vi "measure-6221-SR830(SubVI).vi"(9 "config":refnum<queue>, 11 "错误输入":errorcluster) -> (4 "输出数组":string[](array[string]), 8 "错误输出":errorcluster)   [LabVIEW 2019, in "SubVI.lvlib"]
uses:
  SubVI.lvlib
  config.ctl
  Instrument.ctl
  lib/QDInstrument.dll
  lib/Stanford Research 830/Public/Data/Read (All Parameters).vi
  lib/Stanford Research 830/Stanford Research 830.lvlib
  lib/Keithley 622x/Keithley 622x.lvlib
panel:
  out "输出簇":T1={"initialize"="", "6221"={"6221 Resource"="GPIB0::24::INSTR", "Delta status"=FALSE}, "7001"={"Ch"=FALSE}, "SR830+6221"={"source"=0, "阻抗"=0.0, "量程入 4"=0, "量程入 3"=0, "量程入 2"=0, "量程入 1"=0, "电流"=0.0, "SR830 2"=FALSE, "SR830 3"=FALSE, "SR830 4"=FALSE, "SR830 1"=FALSE, "VISA 1"="", "VISA 2"="", "VISA 3"="", "VISA 4"="", "量程"=enum."量程每次测量会判定"}, "2400"={"2400"=FALSE, "VISA"=""}, "ch"={"ch str"="", "ch1"=FALSE, "ch2"=FALSE, "布尔"=FALSE}, "error"=FALSE, "数据文件路径"=path "", "log"={"log路径"=path "", "log interval"=0.0}, "Instrument"={"335 Resource"="GPIB0::24::INSTR", "Input (0:A)"=0, "Instrument Type"=3, "quantum design"=refnum, "Heater Output (1:1)"=1}} {"Instrument"."Input (0:A)" items=["A", "B"]; "Instrument"."Instrument Type" items=["PPMS", "VersaLab", "DynaCool", "SVSM", "Lakeshore335", "PPMS-Rotate"]; "Instrument"."Heater Output (1:1)" items=["1"=1, "2"=2]; "SR830+6221"."source" items=["SR830 1", "SR830 2", "SR830 3", "SR830 4"]}
  # "(真是通道1，假是通道2)"
  # "(真是通道1，假是通道2)"
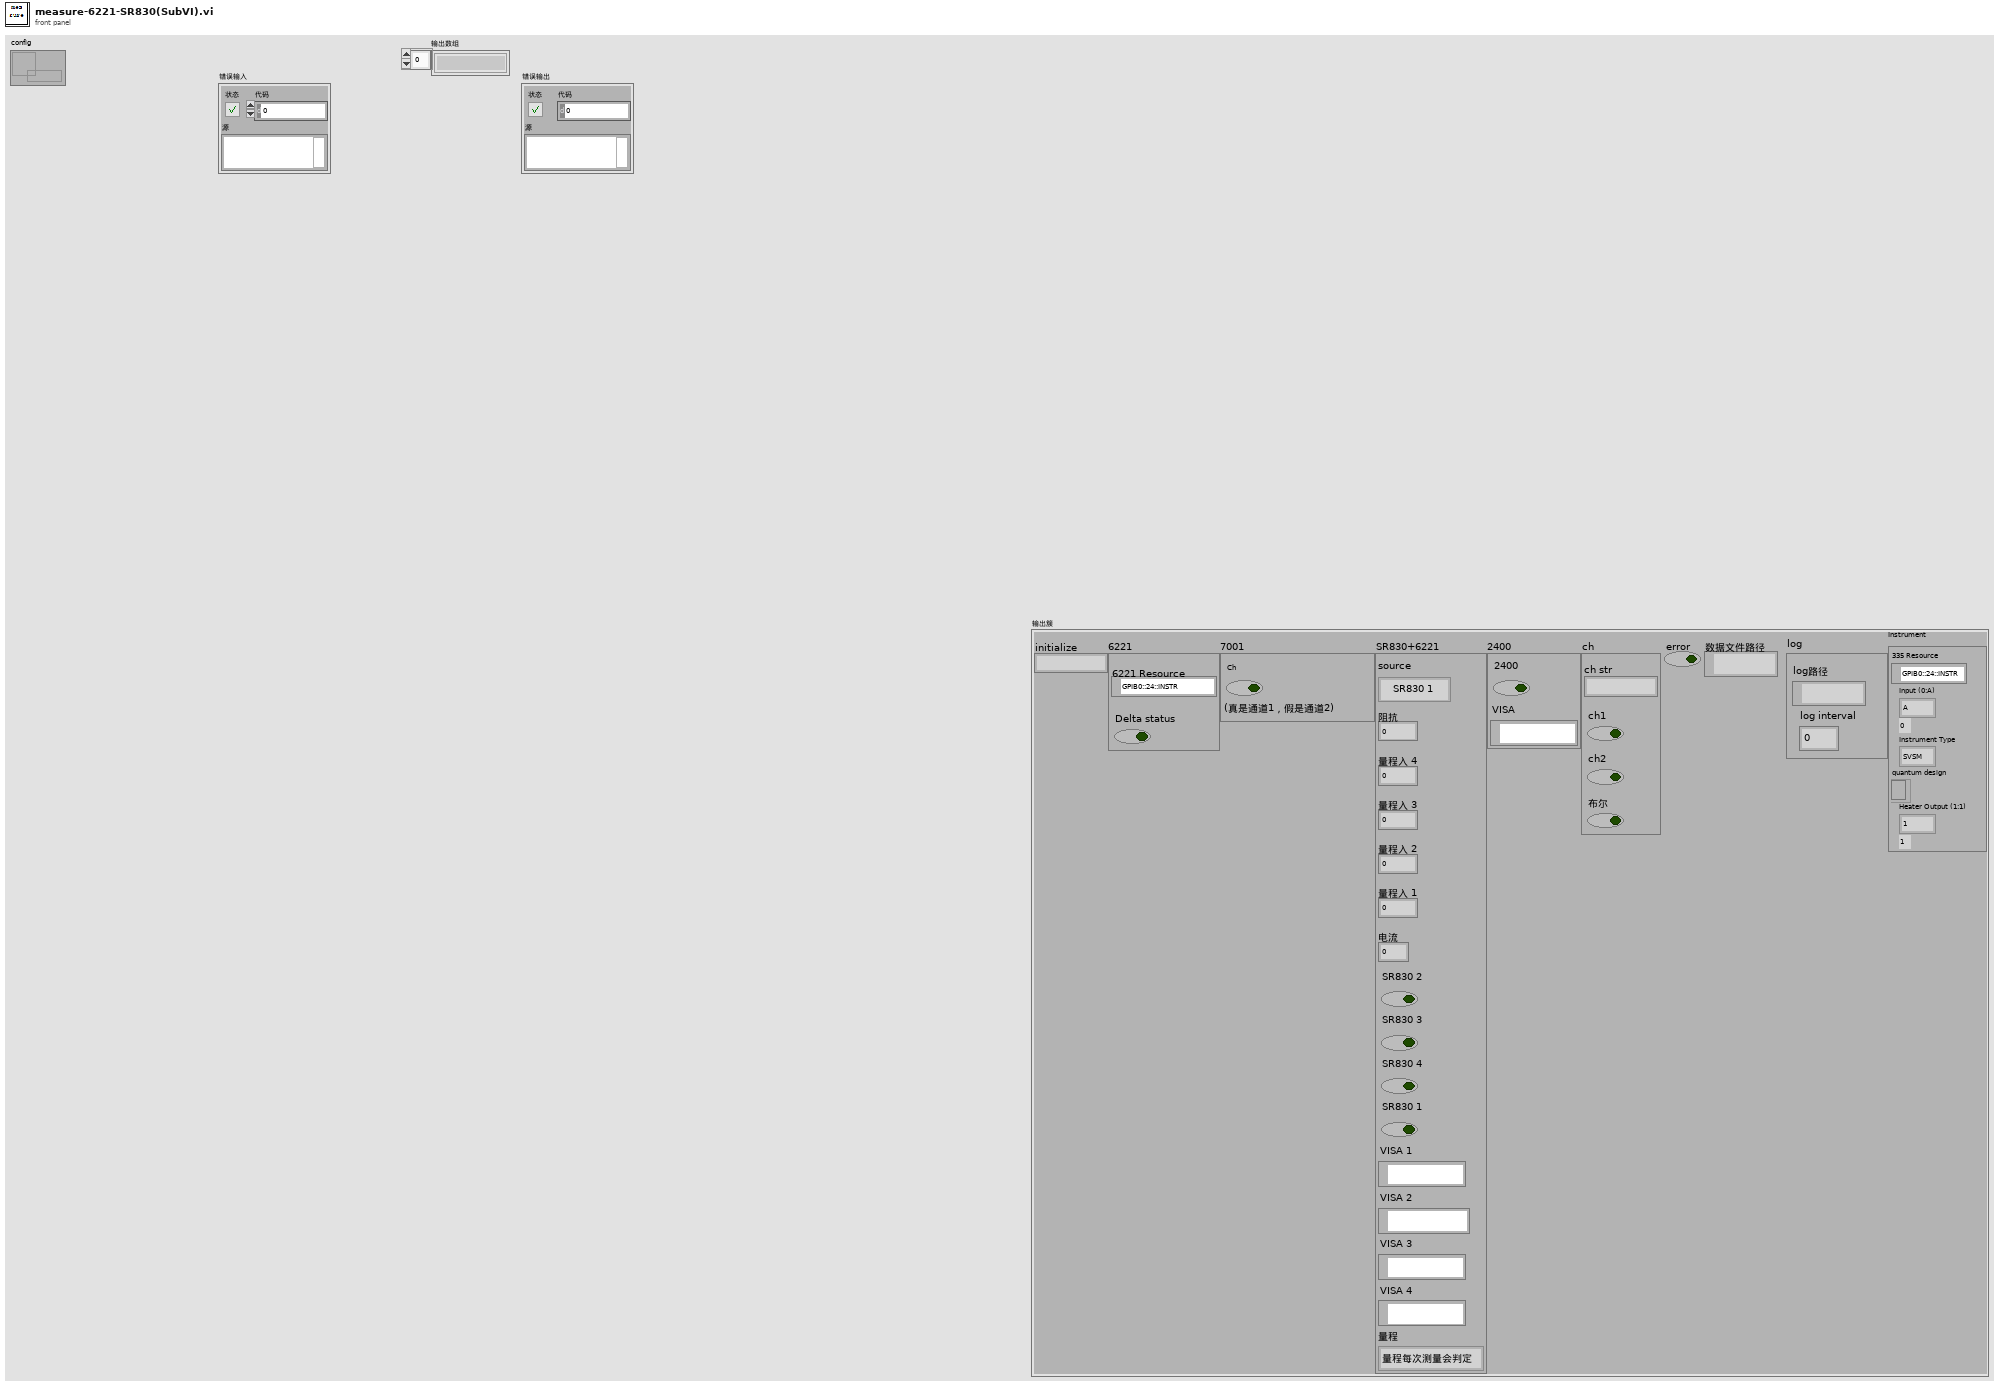
[diagram p1: front panel]
types:
  T1 = typedef "config.ctl" = cluster{"initialize":string, "6221":cluster{"6221 Resource":refnum<visa-resource-name>, "Delta status":bool}, "7001":cluster{"Ch":bool}, "SR830+6221":cluster{"source":u16, "阻抗":dbl, "量程入 4":i32, "量程入 3":i32, "量程入 2":i32, "量程入 1":i32, "电流":dbl, "SR830 2":bool, "SR830 3":bool, "SR830 4":bool, "SR830 1":bool, "VISA 1":refnum<visa-resource-name>, "VISA 2":refnum<visa-resource-name>, "VISA 3":refnum<visa-resource-name>, "VISA 4":refnum<visa-resource-name>, "量程":enum16{"量程每次测量会判定", "量程不变为设定值"}}, "2400":cluster{"2400":bool, "VISA":refnum<visa-resource-name>}, "ch":cluster{"ch str":string, "ch1":bool, "ch2":bool, "布尔":bool}, "error":bool, "数据文件路径":path, "log":cluster{"log路径":path, "log interval":dbl}, "Instrument":T2}
  T2 = typedef "Instrument.ctl" = cluster{"335 Resource":refnum<visa-resource-name>, "Input (0:A)":u16, "Instrument Type":i32, "quantum design":refnum<k24>, "Heater Output (1:1)":u16}
  T3 = cluster{"X-Value":dbl, "Y-Value":dbl, "R-Value":dbl, "Theta-Value":dbl, "Aux In 1 Value":dbl, "Aux In 2 Value":dbl, "Aux In 3 Value":dbl, "Aux In 4 Value":dbl, "Reference Frequency":dbl, "Channel 1 Display":dbl, "Channel 2 Display":dbl}
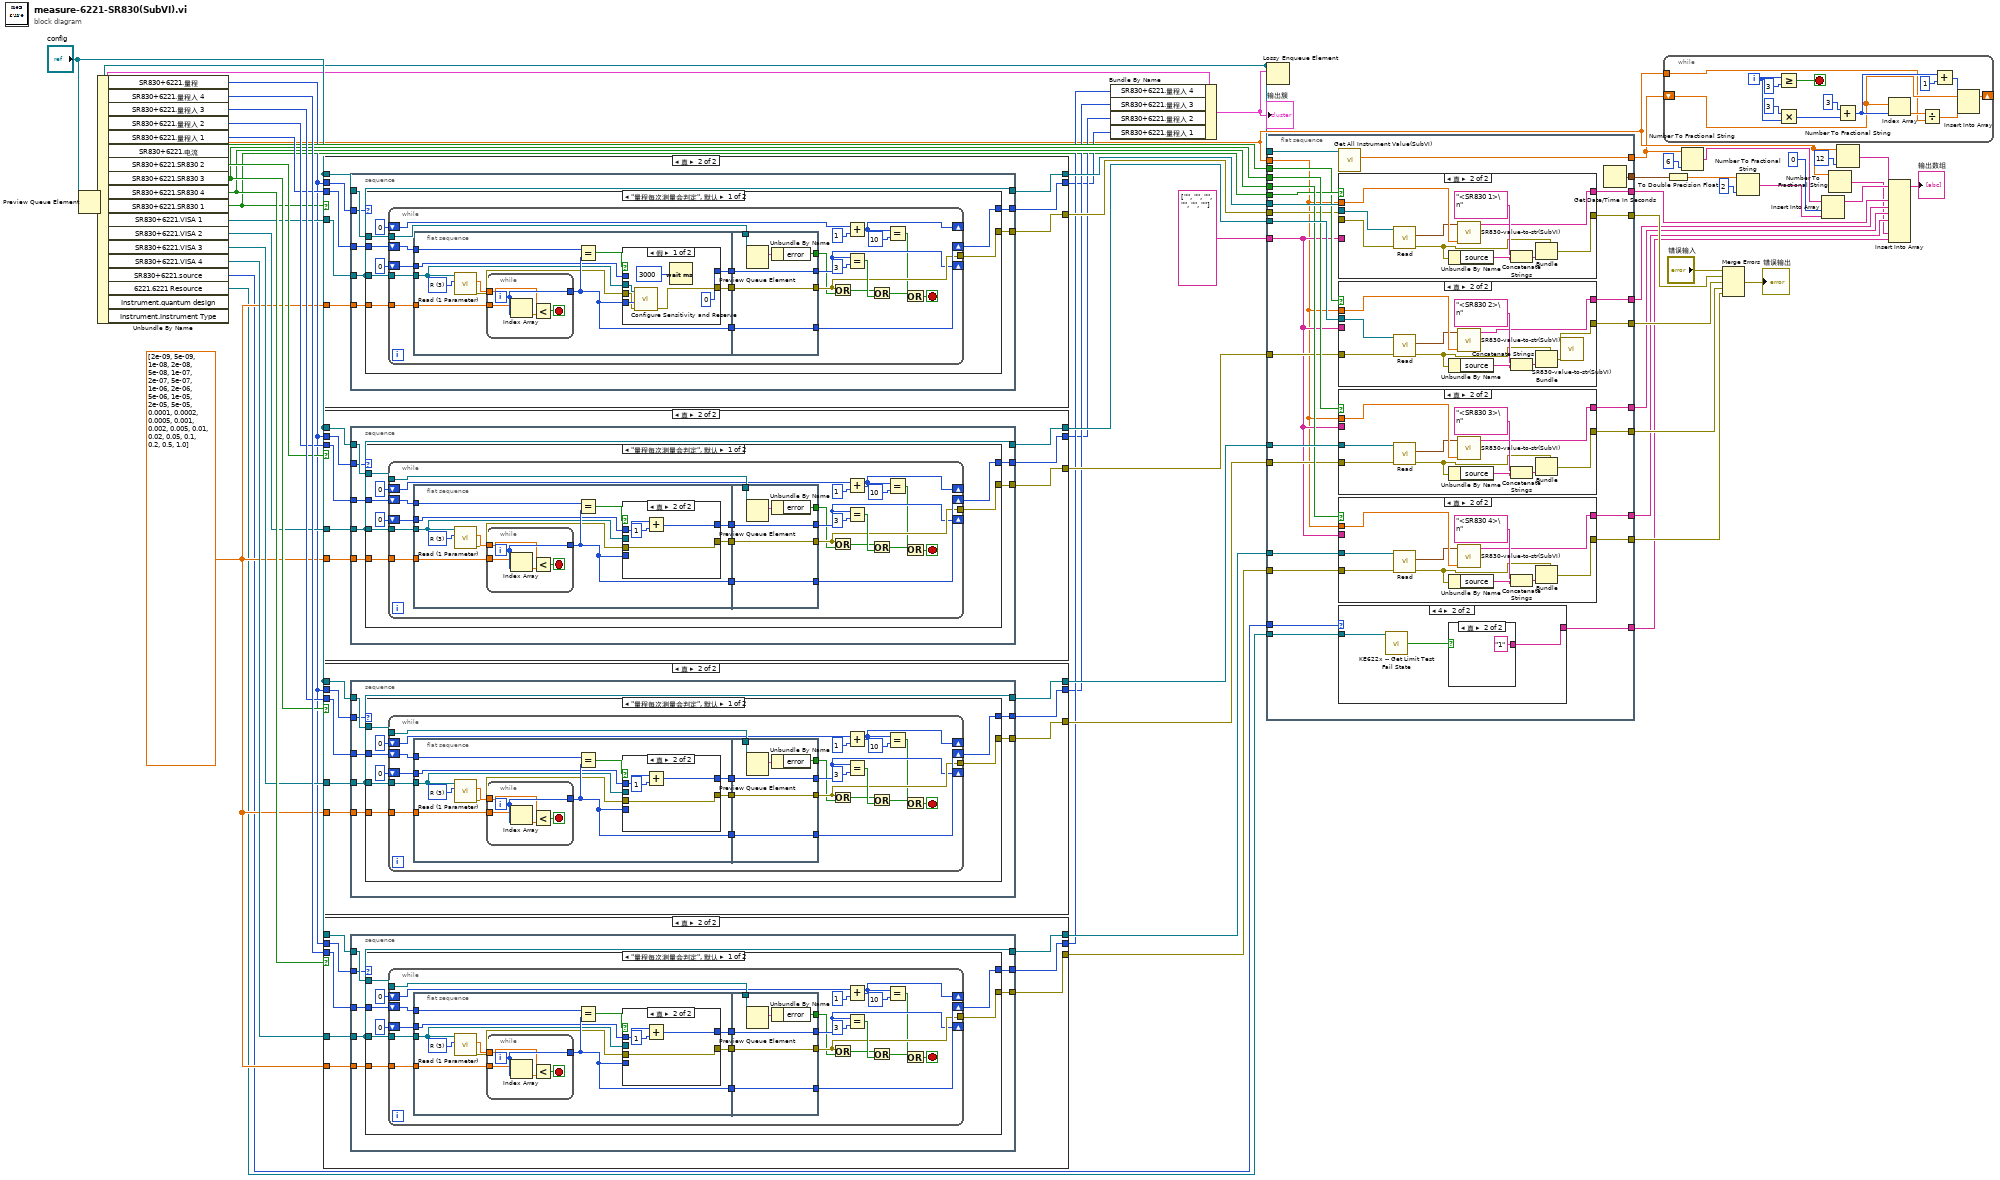
[diagram p0: block diagram]
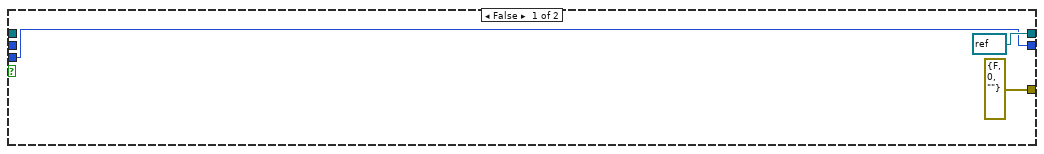
[diagram p2: hidden frame]
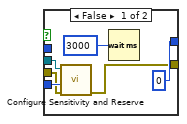
[diagram p3: hidden frame]
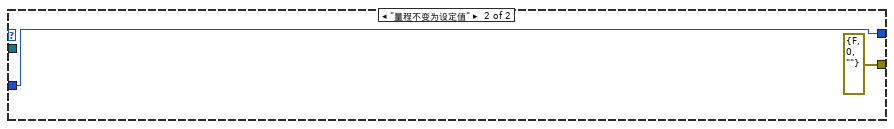
[diagram p4: hidden frame]
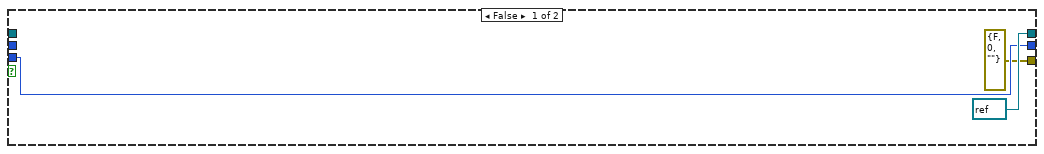
[diagram p5: hidden frame]
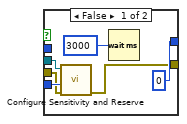
[diagram p6: hidden frame]
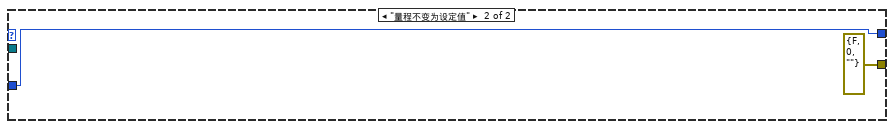
[diagram p7: hidden frame]
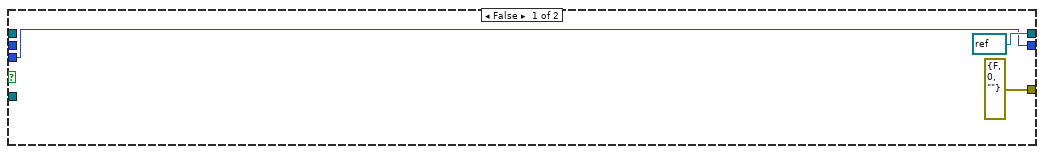
[diagram p8: hidden frame]
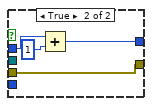
[diagram p9: hidden frame]
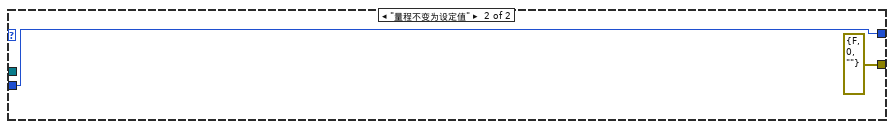
[diagram p10: hidden frame]
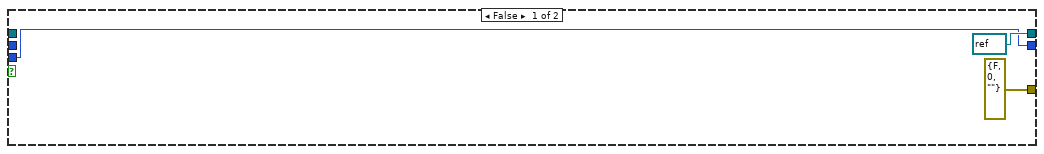
[diagram p11: hidden frame]
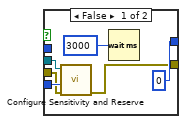
[diagram p12: hidden frame]
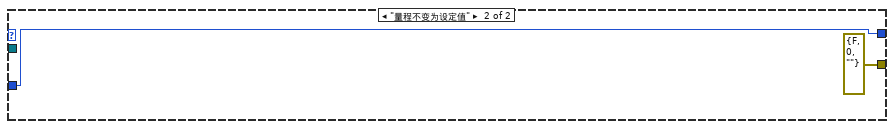
[diagram p13: hidden frame]
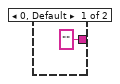
[diagram p14: hidden frame]
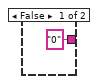
[diagram p15: hidden frame]
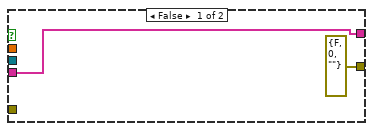
[diagram p16: hidden frame]
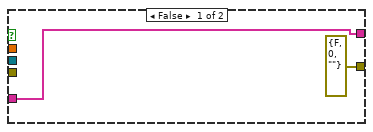
[diagram p17: hidden frame]
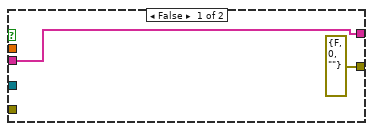
[diagram p18: hidden frame]
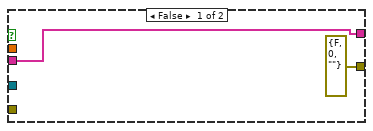
[diagram p19: hidden frame]
diagram:
  w11 = dbl[] [2e-09, 5e-09, 1e-08, 2e-08, 5e-08, 1e-07, 2e-07, 5e-07, 1e-06, 2e-06, 5e-06, 1e-05, 2e-05, 5e-05, 0.0001, 0.0002, 0.0005, 0.001, 0.002, 0.005, 0.01, 0.02, 0.05, 0.1, 0.2, 0.5, 1.0]
  n1 = Preview Queue Element(queue="config") -> (queue out=w2:refnum<queue>, element=w9:T1)  [unwired: 2 in, 2 out]
  n2 = Unbundle By Name(w9) -> ("SR830+6221.量程"=w32:enum16{"量程每次测量会判定", "量程不变为设定值"}, "SR830+6221.量程入 4"=w43:i32, "SR830+6221.量程入 3"=w42:i32, "SR830+6221.量程入 2"=w41:i32, "SR830+6221.量程入 1"=w40:i32, "SR830+6221.电流"=w5:dbl, "SR830+6221.SR830 2"=w39:bool, "SR830+6221.SR830 3"=w38:bool, "SR830+6221.SR830 4"=w37:bool, "SR830+6221.SR830 1"=w19:bool, "SR830+6221.VISA 1"=w36:refnum<visa-resource-name>, "SR830+6221.VISA 2"=w35:refnum<visa-resource-name>, "SR830+6221.VISA 3"=w34:refnum<visa-resource-name>, "SR830+6221.VISA 4"=w33:refnum<visa-resource-name>, "SR830+6221.source"=w7:u16, "6221.6221 Resource"=w6:refnum<visa-resource-name>)  [unwired: 2 out]
  n3 = case shown="真" w19 {
    tunnel: [refnum<visa-resource-name> refnum ("VISA引用句柄输出") w69] -> w56
    tunnel: w32 -> [_ w68]
    tunnel: w36 -> [_ w67]
    tunnel: w40 -> [w60 w66]
    tunnel: [w60 w65] -> w28
    tunnel: "config" -> [_ w64]
    tunnel: [errorcluster {"status"=FALSE, "code"=0, "source"=""} ("error out") w63] -> w53
    tunnel: w11 -> [_ w62]
    frame False {
    }
    frame True {
      n4 = stacked-sequence {
        tunnel: [w75] -> w63
        tunnel: [w71] -> w65
        tunnel: [w73] -> w69
        tunnel: w68 -> [w74]
        tunnel: w64 -> [w76]
        tunnel: w66 -> [w72]
        tunnel: w67 -> [w73]
        tunnel: w62 -> [w70]
        frame #0 {
          n5 = case shown="\"量程每次测量会判定\", 默认" w74 {
            tunnel: [w84 w140] -> w71
            tunnel: w72 -> [w83 w140]
            tunnel: w73 -> [w82 _]
            tunnel: w70 -> [w81 _]
            tunnel: w76 -> [w79 _]
            tunnel: [w78 errorcluster {"status"=FALSE, "code"=0, "source"=""} ("error out")] -> w75
            frame "量程每次测量会判定", Default {
              n6 = while {
                tunnel: w82 -> [w106]
                tunnel: w81 -> [w105]
                shift-right: [w103] -> w84
                shift-left: w83 -> [w102]
                shift-right: [w93] -> _
                shift-left: 0 -> [w101]
                tunnel: w79 -> [w96]
                tunnel: [w95] -> w78
                shift-right: [w86] -> _
                shift-left: 0 -> [w88]
                stop <- w89 stop-if-true
                n7 = flat-sequence {
                  tunnel: w101 -> [w111]
                  tunnel: w102 -> [w112]
                  tunnel: w105 -> [w115]
                  tunnel: w106 -> [w109]
                  tunnel: [w110] -> w99
                  tunnel: [w117] -> w98
                  tunnel: [w107] -> w97
                  tunnel: [w136] -> w95
                  tunnel: [w137] -> w103
                  tunnel: [w138] -> w93
                  tunnel: w99 -> [w138]
                  tunnel: w98 -> [w137]
                  tunnel: w97 -> [w136]
                  tunnel: w96 -> [w135]
                  tunnel: [w133] -> w85
                  frame #0 {
                    w114 = u16 3 items=["X"=1, "Y"=2, "R"=3, "Theta"=4, "Channel 1"=5, "Channel 2"=6, "Aux In 1"=7, "Aux In 2"=8, "Aux In 3"=9, "Aux In 4"=10] ("Parameter (1: X)")
                    n8 = call "Read (1 Parameter).vi"("Parameter (1: X)"=w114, "VISA resource name"=w109) -> ("error out"=w108:errorcluster, "Measurement"=w113:dbl)  [unwired: 7 in, 1 out]
                    n9 = while {
                      tunnel: [w120] -> w117
                      tunnel: w115 -> [w119]
                      tunnel: w113 -> [w118]
                      i -> [w120]
                      stop <- w122 stop-if-true
                      n10 = Index Array(array=w119, index=w120) -> (element=w121:dbl)
                      n11 = Less?(x=w118, y=w121) -> (x < y?=w122:bool)
                    }
                    n12 = Equal?(x=w112, y=w117) -> (x = y?=w116:bool)
                    n13 = case shown="假" w116 {
                      tunnel: w117 -> [w128 _]
                      tunnel: w109 -> [w127 _]
                      tunnel: w111 -> [_ w131]
                      tunnel: [0 w130] -> w110
                      tunnel: w108 -> [w124 w129]
                      tunnel: [w123 w129] -> w107
                      frame False {
                        n14 = call "Configure Sensitivity and Reserve.vi"("error in (no error)"=w124, "Sensitivity (-1: Auto gain)"=w128, "VISA resource name"=w127) -> ("error out"=w123:errorcluster)  [unwired: 7 in, 1 out]
                        n15 = Wait (ms)(milliseconds to wait=u32 3000 ("等待时间（毫秒）")) -> ()  [unwired: 1 out]
                      }
                      frame True {
                        n16 = Add(x=w131, y=1) -> (x+y=w130:i32)
                      }
                    }
                  }
                  frame #1 {
                    n17 = Preview Queue Element(queue=w135) -> (element=w134:T1)  [unwired: 2 in, 3 out]
                    n18 = Unbundle By Name(w134) -> ("error"=w133:bool)
                  }
                }
                n19 = Or(x=w95, y=w85) -> (x .or. y?=w94:bool)
                n20 = Add(x=w88, y=1) -> (x+y=w86:i32)
                n21 = Equal?(x=w93, y=3) -> (x = y?=w100:bool)
                n22 = Or(x=w94, y=w100) -> (x .or. y?=w91:bool)
                n23 = Equal?(x=w86, y=10) -> (x = y?=w90:bool)
                n24 = Or(x=w91, y=w90) -> (x .or. y?=w89:bool)
              }
            }
            frame "量程不变为设定值" {
            }
          }
        }
      }
    }
  }
  n25 = case shown="真" w39 {
    tunnel: [refnum<visa-resource-name> refnum ("VISA引用句柄输出") w151] -> w58
    tunnel: w32 -> [_ w150]
    tunnel: w35 -> [_ w149]
    tunnel: w41 -> [w142 w148]
    tunnel: [w142 w147] -> w29
    tunnel: "config" -> [_ w146]
    tunnel: [errorcluster {"status"=FALSE, "code"=0, "source"=""} ("error out") w145] -> w52
    tunnel: w11 -> [_ w144]
    frame False {
    }
    frame True {
      n26 = stacked-sequence {
        tunnel: [w157] -> w145
        tunnel: [w153] -> w147
        tunnel: [w155] -> w151
        tunnel: w150 -> [w156]
        tunnel: w146 -> [w158]
        tunnel: w148 -> [w154]
        tunnel: w149 -> [w155]
        tunnel: w144 -> [w152]
        frame #0 {
          n27 = case shown="\"量程每次测量会判定\", 默认" w156 {
            tunnel: [w166 w222] -> w153
            tunnel: w154 -> [w165 w222]
            tunnel: w155 -> [w164 _]
            tunnel: w152 -> [w163 _]
            tunnel: w158 -> [w161 _]
            tunnel: [w160 errorcluster {"status"=FALSE, "code"=0, "source"=""} ("error out")] -> w157
            frame "量程每次测量会判定", Default {
              n28 = while {
                tunnel: w164 -> [w188]
                tunnel: w163 -> [w187]
                shift-right: [w185] -> w166
                shift-left: w165 -> [w184]
                shift-right: [w175] -> _
                shift-left: 0 -> [w183]
                tunnel: w161 -> [w178]
                tunnel: [w177] -> w160
                shift-right: [w168] -> _
                shift-left: 0 -> [w170]
                stop <- w171 stop-if-true
                n29 = flat-sequence {
                  tunnel: w183 -> [w193]
                  tunnel: w184 -> [w194]
                  tunnel: w187 -> [w197]
                  tunnel: w188 -> [w191]
                  tunnel: [w192] -> w181
                  tunnel: [w199] -> w180
                  tunnel: [w189] -> w179
                  tunnel: [w218] -> w177
                  tunnel: [w219] -> w185
                  tunnel: [w220] -> w175
                  tunnel: w181 -> [w220]
                  tunnel: w180 -> [w219]
                  tunnel: w179 -> [w218]
                  tunnel: w178 -> [w217]
                  tunnel: [w215] -> w167
                  frame #0 {
                    w196 = u16 3 items=["X"=1, "Y"=2, "R"=3, "Theta"=4, "Channel 1"=5, "Channel 2"=6, "Aux In 1"=7, "Aux In 2"=8, "Aux In 3"=9, "Aux In 4"=10] ("Parameter (1: X)")
                    n30 = call "Read (1 Parameter).vi"("Parameter (1: X)"=w196, "VISA resource name"=w191) -> ("error out"=w190:errorcluster, "Measurement"=w195:dbl)  [unwired: 7 in, 1 out]
                    n31 = while {
                      tunnel: [w202] -> w199
                      tunnel: w197 -> [w201]
                      tunnel: w195 -> [w200]
                      i -> [w202]
                      stop <- w204 stop-if-true
                      n32 = Index Array(array=w201, index=w202) -> (element=w203:dbl)
                      n33 = Less?(x=w200, y=w203) -> (x < y?=w204:bool)
                    }
                    n34 = Equal?(x=w194, y=w199) -> (x = y?=w198:bool)
                    n35 = case shown="真" w198 {
                      tunnel: w199 -> [w210 _]
                      tunnel: w191 -> [w209 _]
                      tunnel: w193 -> [_ w213]
                      tunnel: [0 w212] -> w192
                      tunnel: w190 -> [w206 w211]
                      tunnel: [w205 w211] -> w189
                      frame False {
                        n36 = call "Configure Sensitivity and Reserve.vi"("error in (no error)"=w206, "Sensitivity (-1: Auto gain)"=w210, "VISA resource name"=w209) -> ("error out"=w205:errorcluster)  [unwired: 7 in, 1 out]
                        n37 = Wait (ms)(milliseconds to wait=u32 3000 ("等待时间（毫秒）")) -> ()  [unwired: 1 out]
                      }
                      frame True {
                        n38 = Add(x=w213, y=1) -> (x+y=w212:i32)
                      }
                    }
                  }
                  frame #1 {
                    n39 = Preview Queue Element(queue=w217) -> (element=w216:T1)  [unwired: 2 in, 3 out]
                    n40 = Unbundle By Name(w216) -> ("error"=w215:bool)
                  }
                }
                n41 = Or(x=w177, y=w167) -> (x .or. y?=w176:bool)
                n42 = Add(x=w170, y=1) -> (x+y=w168:i32)
                n43 = Equal?(x=w175, y=3) -> (x = y?=w182:bool)
                n44 = Or(x=w176, y=w182) -> (x .or. y?=w173:bool)
                n45 = Equal?(x=w168, y=10) -> (x = y?=w172:bool)
                n46 = Or(x=w173, y=w172) -> (x .or. y?=w171:bool)
              }
            }
            frame "量程不变为设定值" {
            }
          }
        }
      }
    }
  }
  n47 = case shown="真" w38 {
    tunnel: [refnum<visa-resource-name> refnum ("VISA引用句柄输出") w233] -> w55
    tunnel: w32 -> [_ w232]
    tunnel: w34 -> [_ w231]
    tunnel: w42 -> [w224 w230]
    tunnel: [w224 w229] -> w30
    tunnel: "config" -> [_ w228]
    tunnel: [errorcluster {"status"=FALSE, "code"=0, "source"=""} ("error out") w227] -> w51
    tunnel: w11 -> [_ w226]
    frame False {
    }
    frame True {
      n48 = stacked-sequence {
        tunnel: [w239] -> w227
        tunnel: [w235] -> w229
        tunnel: [w237] -> w233
        tunnel: w232 -> [w238]
        tunnel: w228 -> [w240]
        tunnel: w230 -> [w236]
        tunnel: w231 -> [w237]
        tunnel: w226 -> [w234]
        frame #0 {
          n49 = case shown="\"量程每次测量会判定\", 默认" w238 {
            tunnel: [w248 w304] -> w235
            tunnel: w236 -> [w247 w304]
            tunnel: w237 -> [w246 _]
            tunnel: w234 -> [w245 _]
            tunnel: w240 -> [w243 _]
            tunnel: [w242 errorcluster {"status"=FALSE, "code"=0, "source"=""} ("error out")] -> w239
            frame "量程每次测量会判定", Default {
              n50 = while {
                tunnel: w246 -> [w270]
                tunnel: w245 -> [w269]
                shift-right: [w267] -> w248
                shift-left: w247 -> [w266]
                shift-right: [w257] -> _
                shift-left: 0 -> [w265]
                tunnel: w243 -> [w260]
                tunnel: [w259] -> w242
                shift-right: [w250] -> _
                shift-left: 0 -> [w252]
                stop <- w253 stop-if-true
                n51 = flat-sequence {
                  tunnel: w265 -> [w275]
                  tunnel: w266 -> [w276]
                  tunnel: w269 -> [w279]
                  tunnel: w270 -> [w273]
                  tunnel: [w274] -> w263
                  tunnel: [w281] -> w262
                  tunnel: [w271] -> w261
                  tunnel: [w300] -> w259
                  tunnel: [w301] -> w267
                  tunnel: [w302] -> w257
                  tunnel: w263 -> [w302]
                  tunnel: w262 -> [w301]
                  tunnel: w261 -> [w300]
                  tunnel: w260 -> [w299]
                  tunnel: [w297] -> w249
                  frame #0 {
                    w278 = u16 3 items=["X"=1, "Y"=2, "R"=3, "Theta"=4, "Channel 1"=5, "Channel 2"=6, "Aux In 1"=7, "Aux In 2"=8, "Aux In 3"=9, "Aux In 4"=10] ("Parameter (1: X)")
                    n52 = call "Read (1 Parameter).vi"("Parameter (1: X)"=w278, "VISA resource name"=w273) -> ("error out"=w272:errorcluster, "Measurement"=w277:dbl)  [unwired: 7 in, 1 out]
                    n53 = while {
                      tunnel: [w284] -> w281
                      tunnel: w279 -> [w283]
                      tunnel: w277 -> [w282]
                      i -> [w284]
                      stop <- w286 stop-if-true
                      n54 = Index Array(array=w283, index=w284) -> (element=w285:dbl)
                      n55 = Less?(x=w282, y=w285) -> (x < y?=w286:bool)
                    }
                    n56 = Equal?(x=w276, y=w281) -> (x = y?=w280:bool)
                    n57 = case shown="真" w280 {
                      tunnel: w281 -> [w292 _]
                      tunnel: w273 -> [w291 _]
                      tunnel: w275 -> [_ w295]
                      tunnel: [0 w294] -> w274
                      tunnel: w272 -> [w288 w293]
                      tunnel: [w287 w293] -> w271
                      frame False {
                        n58 = call "Configure Sensitivity and Reserve.vi"("error in (no error)"=w288, "Sensitivity (-1: Auto gain)"=w292, "VISA resource name"=w291) -> ("error out"=w287:errorcluster)  [unwired: 7 in, 1 out]
                        n59 = Wait (ms)(milliseconds to wait=u32 3000 ("等待时间（毫秒）")) -> ()  [unwired: 1 out]
                      }
                      frame True {
                        n60 = Add(x=w295, y=1) -> (x+y=w294:i32)
                      }
                    }
                  }
                  frame #1 {
                    n61 = Preview Queue Element(queue=w299) -> (element=w298:T1)  [unwired: 2 in, 3 out]
                    n62 = Unbundle By Name(w298) -> ("error"=w297:bool)
                  }
                }
                n63 = Or(x=w259, y=w249) -> (x .or. y?=w258:bool)
                n64 = Add(x=w252, y=1) -> (x+y=w250:i32)
                n65 = Equal?(x=w257, y=3) -> (x = y?=w264:bool)
                n66 = Or(x=w258, y=w264) -> (x .or. y?=w255:bool)
                n67 = Equal?(x=w250, y=10) -> (x = y?=w254:bool)
                n68 = Or(x=w255, y=w254) -> (x .or. y?=w253:bool)
              }
            }
            frame "量程不变为设定值" {
            }
          }
        }
      }
    }
  }
  n69 = case shown="真" w37 {
    tunnel: [refnum<visa-resource-name> refnum ("VISA引用句柄输出") w315] -> w57
    tunnel: w32 -> [_ w314]
    tunnel: w33 -> [_ w313]
    tunnel: [w306 w312] -> w31
    tunnel: w43 -> [w306 w311]
    tunnel: "config" -> [_ w310]
    tunnel: [errorcluster {"status"=FALSE, "code"=0, "source"=""} ("error out") w309] -> w50
    tunnel: w11 -> [_ w308]
    frame False {
    }
    frame True {
      n70 = stacked-sequence {
        tunnel: [w321] -> w309
        tunnel: [w317] -> w312
        tunnel: [w319] -> w315
        tunnel: w314 -> [w320]
        tunnel: w310 -> [w322]
        tunnel: w311 -> [w318]
        tunnel: w313 -> [w319]
        tunnel: w308 -> [w316]
        frame #0 {
          n71 = case shown="\"量程每次测量会判定\", 默认" w320 {
            tunnel: [w330 w386] -> w317
            tunnel: w318 -> [w329 w386]
            tunnel: w319 -> [w328 _]
            tunnel: w316 -> [w327 _]
            tunnel: w322 -> [w325 _]
            tunnel: [w324 errorcluster {"status"=FALSE, "code"=0, "source"=""} ("error out")] -> w321
            frame "量程每次测量会判定", Default {
              n72 = while {
                tunnel: w328 -> [w352]
                tunnel: w327 -> [w351]
                shift-right: [w349] -> w330
                shift-left: w329 -> [w348]
                shift-right: [w339] -> _
                shift-left: 0 -> [w347]
                tunnel: w325 -> [w342]
                tunnel: [w341] -> w324
                shift-right: [w332] -> _
                shift-left: 0 -> [w334]
                stop <- w335 stop-if-true
                n73 = flat-sequence {
                  tunnel: w347 -> [w357]
                  tunnel: w348 -> [w358]
                  tunnel: w351 -> [w361]
                  tunnel: w352 -> [w355]
                  tunnel: [w356] -> w345
                  tunnel: [w363] -> w344
                  tunnel: [w353] -> w343
                  tunnel: [w382] -> w341
                  tunnel: [w383] -> w349
                  tunnel: [w384] -> w339
                  tunnel: w345 -> [w384]
                  tunnel: w344 -> [w383]
                  tunnel: w343 -> [w382]
                  tunnel: w342 -> [w381]
                  tunnel: [w379] -> w331
                  frame #0 {
                    w360 = u16 3 items=["X"=1, "Y"=2, "R"=3, "Theta"=4, "Channel 1"=5, "Channel 2"=6, "Aux In 1"=7, "Aux In 2"=8, "Aux In 3"=9, "Aux In 4"=10] ("Parameter (1: X)")
                    n74 = call "Read (1 Parameter).vi"("Parameter (1: X)"=w360, "VISA resource name"=w355) -> ("error out"=w354:errorcluster, "Measurement"=w359:dbl)  [unwired: 7 in, 1 out]
                    n75 = while {
                      tunnel: [w366] -> w363
                      tunnel: w361 -> [w365]
                      tunnel: w359 -> [w364]
                      i -> [w366]
                      stop <- w368 stop-if-true
                      n76 = Index Array(array=w365, index=w366) -> (element=w367:dbl)
                      n77 = Less?(x=w364, y=w367) -> (x < y?=w368:bool)
                    }
                    n78 = Equal?(x=w358, y=w363) -> (x = y?=w362:bool)
                    n79 = case shown="真" w362 {
                      tunnel: w363 -> [w374 _]
                      tunnel: w355 -> [w373 _]
                      tunnel: w357 -> [_ w377]
                      tunnel: [0 w376] -> w356
                      tunnel: w354 -> [w370 w375]
                      tunnel: [w369 w375] -> w353
                      frame False {
                        n80 = call "Configure Sensitivity and Reserve.vi"("error in (no error)"=w370, "Sensitivity (-1: Auto gain)"=w374, "VISA resource name"=w373) -> ("error out"=w369:errorcluster)  [unwired: 7 in, 1 out]
                        n81 = Wait (ms)(milliseconds to wait=u32 3000 ("等待时间（毫秒）")) -> ()  [unwired: 1 out]
                      }
                      frame True {
                        n82 = Add(x=w377, y=1) -> (x+y=w376:i32)
                      }
                    }
                  }
                  frame #1 {
                    n83 = Preview Queue Element(queue=w381) -> (element=w380:T1)  [unwired: 2 in, 3 out]
                    n84 = Unbundle By Name(w380) -> ("error"=w379:bool)
                  }
                }
                n85 = Or(x=w341, y=w331) -> (x .or. y?=w340:bool)
                n86 = Add(x=w334, y=1) -> (x+y=w332:i32)
                n87 = Equal?(x=w339, y=3) -> (x = y?=w346:bool)
                n88 = Or(x=w340, y=w346) -> (x .or. y?=w337:bool)
                n89 = Equal?(x=w332, y=10) -> (x = y?=w336:bool)
                n90 = Or(x=w337, y=w336) -> (x .or. y?=w335:bool)
              }
            }
            frame "量程不变为设定值" {
            }
          }
        }
      }
    }
  }
  n91 = Bundle By Name(cluster=w9, "SR830+6221.量程入 4"=w31, "SR830+6221.量程入 3"=w30, "SR830+6221.量程入 2"=w29, "SR830+6221.量程入 1"=w28) -> (w8:T1)
  "输出簇" <- w8
  n92 = Lossy Enqueue Element(queue=w2, element=w8) -> ()  [unwired: 1 in, 4 out]
  n93 = flat-sequence {
    tunnel: [w414] -> w54
    tunnel: w58 -> [w413]
    tunnel: w56 -> [w412]
    tunnel: w57 -> [w411]
    tunnel: w55 -> [w410]
    tunnel: w38 -> [w409]
    tunnel: w37 -> [w408]
    tunnel: w19 -> [w407]
    tunnel: w39 -> [w406]
    tunnel: w53 -> [w405]
    tunnel: w52 -> [w404]
    tunnel: w51 -> [w403]
    tunnel: w50 -> [w402]
    tunnel: [w401] -> w49
    tunnel: [w400] -> w48
    tunnel: [w399] -> w47
    tunnel: [w398] -> w46
    tunnel: [w397] -> w18
    tunnel: [w396] -> w17
    tunnel: [w395] -> w16
    tunnel: w5 -> [w389]
    tunnel: [w394] -> w15
    tunnel: string[] ["", "", "", "", "", ""] ("数组") -> [w390]
    tunnel: [w393] -> w4
    tunnel: w7 -> [w392]
    tunnel: w6 -> [w391]
    tunnel: w2 -> [w388]
    tunnel: [w387] -> w1
    frame #0 {
      n94 = call "Get All Instrument Value(SubVI).vi"("队列输入"=w388) -> ("数组"=w387:dbl[])  [unwired: 10 in]
      n95 = case shown="真" w407 {
        tunnel: w412 -> [_ w444]
        tunnel: w405 -> [_ w443]
        tunnel: [errorcluster {"status"=FALSE, "code"=0, "source"=""} ("error out") w438] -> w401
        tunnel: w389 -> [_ w437]
        tunnel: [w433 w435] -> w397
        tunnel: w390 -> [w433 _]
        frame False {
        }
        frame True {
          n96 = call-poly "Read.vi"("error in (no error)"=w443, "VISA resource name"=w444) -> ("error out"=w439:errorcluster, "Parameter Values"=w436:T3)  [unwired: 7 in, 1 out]
          n97 = Unbundle By Name(w439) -> ("source"=w441:string)
          n98 = call "SR830-value-to-str(SubVI).vi"("电流"=w437, "Parameter Values"=w436) -> ("数组"=w435:string[])  [unwired: 9 in]
          n99 = Concatenate Strings("<SR830 1>\n", w441) -> (w440:string)
          n100 = Bundle(cluster=w439, "source"=w440) -> (w438:errorcluster)  [unwired: 2 in]
        }
      }
      n101 = case shown="真" w406 {
        tunnel: w413 -> [_ w432]
        tunnel: w404 -> [_ w431]
        tunnel: [errorcluster {"status"=FALSE, "code"=0, "source"=""} ("error out") w426] -> w399
        tunnel: w389 -> [_ w425]
        tunnel: [w421 w423] -> w396
        tunnel: w390 -> [w421 _]
        frame False {
        }
        frame True {
          n102 = call-poly "Read.vi"("error in (no error)"=w431, "VISA resource name"=w432) -> ("error out"=w427:errorcluster, "Parameter Values"=w424:T3)  [unwired: 7 in, 1 out]
          n103 = Unbundle By Name(w427) -> ("source"=w429:string)
          n104 = call "SR830-value-to-str(SubVI).vi"("电流"=w425, "Parameter Values"=w424) -> ("数组"=w423:string[])  [unwired: 9 in]
          n105 = Concatenate Strings("<SR830 2>\n", w429) -> (w428:string)
          n106 = Bundle(cluster=w427, "source"=w428) -> (w426:errorcluster)  [unwired: 2 in]
          n107 = call "SR830-value-to-str(SubVI).vi"() -> ()  [unwired: 11 in, 1 out]
        }
      }
      n108 = case shown="真" w409 {
        tunnel: w410 -> [_ w468]
        tunnel: w403 -> [_ w467]
        tunnel: [errorcluster {"status"=FALSE, "code"=0, "source"=""} ("error out") w462] -> w400
        tunnel: w389 -> [_ w461]
        tunnel: [w457 w459] -> w395
        tunnel: w390 -> [w457 _]
        frame False {
        }
        frame True {
          n109 = call-poly "Read.vi"("error in (no error)"=w467, "VISA resource name"=w468) -> ("error out"=w463:errorcluster, "Parameter Values"=w460:T3)  [unwired: 7 in, 1 out]
          n110 = Unbundle By Name(w463) -> ("source"=w465:string)
          n111 = call "SR830-value-to-str(SubVI).vi"("电流"=w461, "Parameter Values"=w460) -> ("数组"=w459:string[])  [unwired: 9 in]
          n112 = Concatenate Strings("<SR830 3>\n", w465) -> (w464:string)
          n113 = Bundle(cluster=w463, "source"=w464) -> (w462:errorcluster)  [unwired: 2 in]
        }
      }
      n114 = case shown="真" w408 {
        tunnel: w411 -> [_ w456]
        tunnel: w402 -> [_ w455]
        tunnel: [errorcluster {"status"=FALSE, "code"=0, "source"=""} ("error out") w450] -> w398
        tunnel: w389 -> [_ w449]
        tunnel: [w445 w447] -> w394
        tunnel: w390 -> [w445 _]
        frame False {
        }
        frame True {
          n115 = call-poly "Read.vi"("error in (no error)"=w455, "VISA resource name"=w456) -> ("error out"=w451:errorcluster, "Parameter Values"=w448:T3)  [unwired: 7 in, 1 out]
          n116 = Unbundle By Name(w451) -> ("source"=w453:string)
          n117 = call "SR830-value-to-str(SubVI).vi"("电流"=w449, "Parameter Values"=w448) -> ("数组"=w447:string[])  [unwired: 9 in]
          n118 = Concatenate Strings("<SR830 4>\n", w453) -> (w452:string)
          n119 = Bundle(cluster=w451, "source"=w452) -> (w450:errorcluster)  [unwired: 2 in]
        }
      }
      n120 = case shown="4" w392 {
        tunnel: ["" w417] -> w393
        tunnel: w391 -> [_ w416]
        frame 0, Default {
        }
        frame 4 {
          n121 = call "KE622x -- Get Limit Test Fail State.vi"("Resource In"=w416) -> ("Limit Test Failed (Compliance)?"=w418:bool)  [unwired: 12 in, 2 out]
          n122 = case shown="真" w418 {
            tunnel: ["0" "1"] -> w417
            frame False {
            }
            frame True {
            }
          }
        }
      }
      n123 = Get Date/Time In Seconds() -> (seconds since 1Jan1904=w414:timestamp)
    }
  }
  n124 = while {
    shift-right: [w477] -> _
    shift-left: w1 -> [w471]
    tunnel: w5 -> [w469]
    i -> [w470]
    stop <- w478 stop-if-true
    n125 = Greater Or Equal?(x=w470, y=3) -> (x >= y?=w478:bool)
    n126 = Multiply(x=3, y=w470) -> (x*y=w480:i32)
    n127 = Add(x=3 ("索引"), y=w480) -> (x+y=w476:i32)
    n128 = Index Array(array=w471, index=w476) -> (element=w473:dbl)
    n129 = Divide(x=w473, y=w469) -> (x/y=w472:dbl)
    n130 = Add(x=w476, y=1) -> (x+y=w474:i32)
    n131 = Insert Into Array(array=w471, index=w474, new element=w472) -> (w477:dbl[])
  }
  n132 = To Double Precision Float(number=w54) -> (double precision float=w24:dbl)
  n133 = Number To Fractional String(number=w1, precision (6)=i16 6 ("精度(6)")) -> (F-format string=w26:string[])  [unwired: 2 in]
  n134 = Merge Errors("错误输入", w49, w47, w48, w46) -> (→"错误输出":errorcluster)
  n135 = Number To Fractional String(number=w24, precision (6)=i16 2 ("精度(6)")) -> (F-format string=w22:string)  [unwired: 2 in]
  n136 = Insert Into Array(array=w26, index=0 ("索引"), new element=w22) -> (w21:string[])
  n137 = Number To Fractional String(number=w5) -> (F-format string=w3:string)  [unwired: 3 in]
  n138 = Number To Fractional String(number=w5, precision (6)=i16 12 ("精度(6)")) -> (F-format string=w12:string)  [unwired: 2 in]
  n139 = Insert Into Array(array=w21, new element #1=w18, new element #2=w17, new element #3=w16, new element #4=w15, new element #5=w12, new element #6=w3, new element #7=w4) -> (→"输出数组":string[])  [unwired: 1 in]
